vi "multiD.vi"(8 "Time Interval Between Repeats mS)":T1 step=2, 9 "Number of repetitions":u16, 10 "Array":T2[](array[typedef]) {"Number Z Slices" min=1 step=1; "Piezo End (µm)" min=0.0 max=100.0; "Piezo Start (µm)" min=0.0 max=100.0; "Beam @ max Z" min=-10.0 max=10.0; "Beam @ min Z" min=-10.0 max=10.0; "Tuneable Lens 2" min=0.0 max=3.0 step=0.0001; "Tuneable Lens 1" min=0.0 max=3.0 step=0.0001; "Scan Mirror Position 2" min=-10.0 max=10.0; "Scan Mirror Position 1" min=-10.0 max=10.0; "Scan Mirror Amplitude" min=-10.0 max=10.0; "Scan Mirror Min" min=-10.0 max=10.0; "Scan Mirror Max" min=-10.0 max=10.0; "Sweep Interval (µS)" step=2; "Sweep Time (µS)" step=2}) -> ()   [LabVIEW 2013]
uses:
  Laser.ctl
  Time_microseconds.ctl
  Phase_Shift.ctl
  Mirror_Voltage.ctl
  Z_Offset.ctl
  Gain.ctl
  Tuneable_Lens_Numeric_Control.ctl
  Piezo_micrometres.ctl
  Microscope_Settings.ctl
  waveforms.ctl
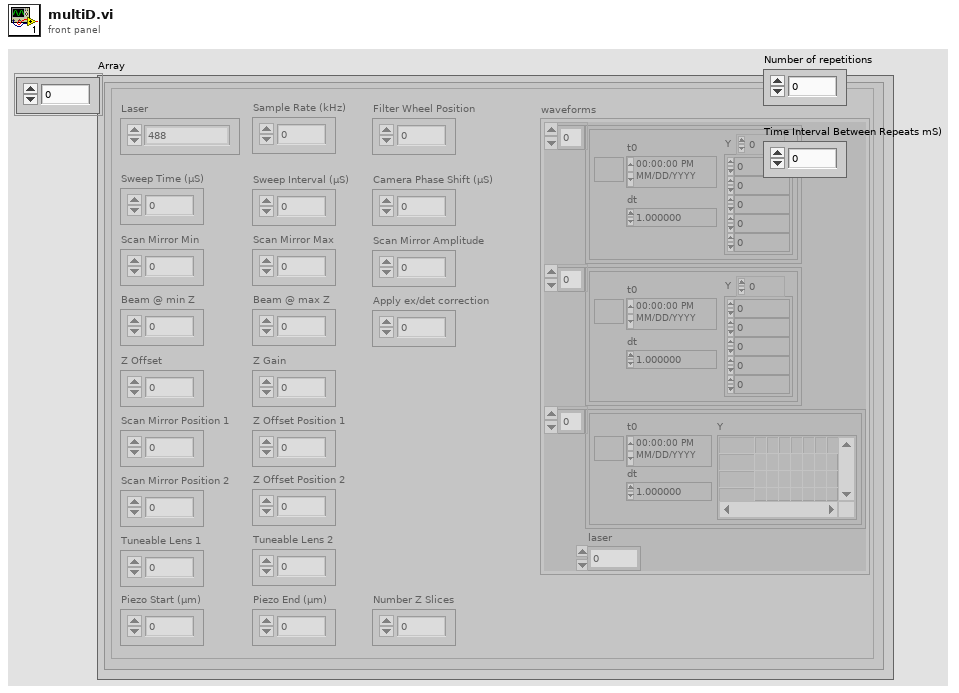
[diagram p1: front panel]
types:
  T1 = typedef "Time_microseconds.ctl" = u32
  T2 = typedef "Microscope_Settings.ctl" = cluster{"Laser":T3, "Sweep Time (µS)":T1, "Sweep Interval (µS)":T1, "Sample Rate (kHz)":dbl, "Camera Phase Shift (µS)":T4, "Scan Mirror Max":T5, "Scan Mirror Min":T5, "Scan Mirror Amplitude":T5, "Z Offset":T6, "Z Gain":T7, "Scan Mirror Position 1":T5, "Z Offset Position 1":T6, "Scan Mirror Position 2":T5, "Z Offset Position 2":T6, "Tuneable Lens 1":T8, "Tuneable Lens 2":T8, "Beam @ min Z":T5, "Beam @ max Z":T5, "Piezo Start (µm)":T9, "Piezo End (µm)":T9, "Number Z Slices":i16, "Filter Wheel Position":i32, "Apply ex/det correction":u16, "waveforms":T10}
  T3 = typedef "Laser.ctl" = enum16{"488", "561"}
  T4 = typedef "Phase_Shift.ctl" = i32
  T5 = typedef "Mirror_Voltage.ctl" = dbl
  T6 = typedef "Z_Offset.ctl" = dbl
  T7 = typedef "Gain.ctl" = dbl
  T8 = typedef "Tuneable_Lens_Numeric_Control.ctl" = dbl
  T9 = typedef "Piezo_micrometres.ctl" = dbl
  T10 = typedef "waveforms.ctl" = cluster{waveform(dbl)[], waveform(dbl)[], digitalwaveform[], "laser":i32}
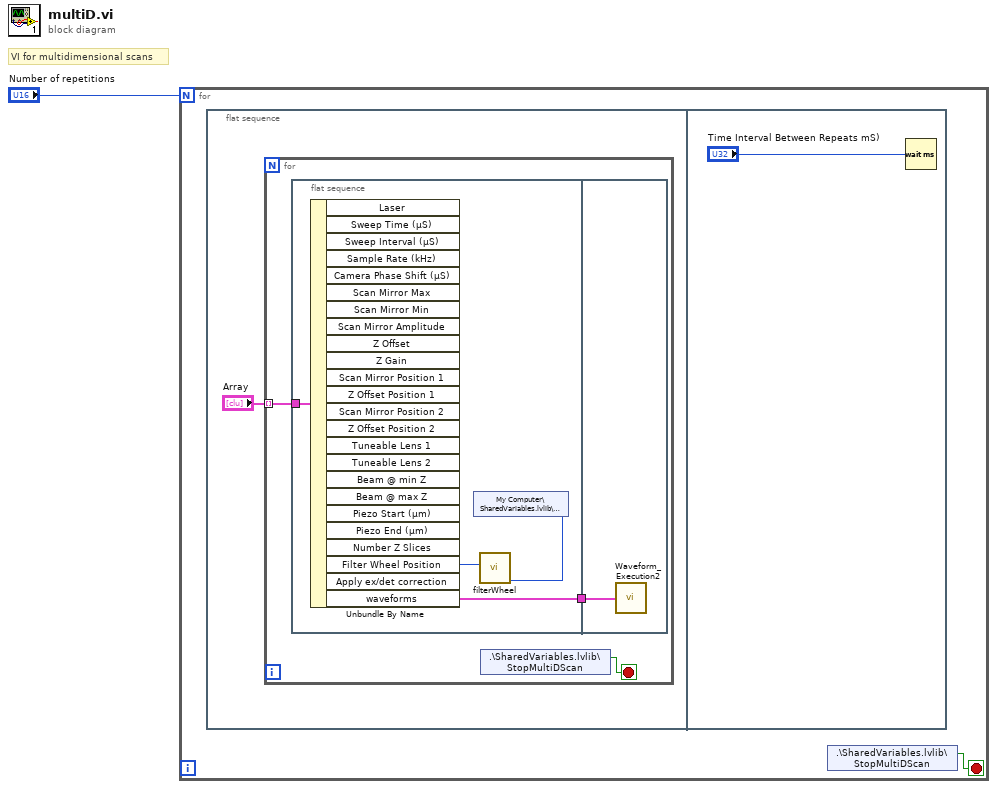
[diagram p0: block diagram]
diagram:
  # "VI for multidimensional scans"
  n1 = for {
    N: "Number of repetitions" -> [_]
    stop <- w2 stop-if-true
    n2 = flat-sequence {
      frame #0 {
        n3 = for {
          tunnel: "Array" -> [w5] mode=indexing
          stop <- w6 stop-if-true
          n4 = flat-sequence {
            tunnel: w5 -> [w10]
            tunnel: [w8] -> w4
            tunnel: w4 -> [w11]
            frame #0 {
              n5 = Unbundle By Name(w10) -> ("Filter Wheel Position"=w9:i32, "waveforms"=w8:T10)  [unwired: 22 out]
              n6 = shared-variable "My Computer\\SharedVariables.lvlib\\COMport"() -> (w7:i32)  [unwired: 1 in, 1 out]
              n7 = call "filterWheel.vi"("serial  port"=w7, "position"=w9) -> ()  [unwired: 10 in]
            }
            frame #1 {
              n8 = call "Waveform_Execution2.vi"("output cluster"=w11) -> ()  [unwired: 3 in]
            }
          }
          n9 = shared-variable ".\\SharedVariables.lvlib\\StopMultiDScan"() -> (w6:bool)  [unwired: 1 in, 1 out]
        }
      }
      frame #1 {
        n10 = Wait (ms)(milliseconds to wait="Time Interval Between Repeats mS)") -> ()  [unwired: 1 out]
      }
    }
    n11 = shared-variable ".\\SharedVariables.lvlib\\StopMultiDScan"() -> (w2:bool)  [unwired: 1 in, 1 out]
  }
